vi "Get All Combinations.vi"(11 "Game Board in":refnum<class "Game Board.lvclass">) -> (3 "Game Board out":refnum<class "Game Board.lvclass">)   [LabVIEW 2024, in "Game Board.lvclass"]
doc: "MIT Licence\nCopyright (c) 2024 David Grollier"
uses:
  Game Board.lvclass
  Combinations Collision.ctl
  Collision/Collision.lvclass
  Game Board.lvclass/Game Board.ctl
  Game Board Component/Movable/Movable.lvclass
  Game Board Component/Game Board Component.lvclass
panel:
  out "appended array":string[][](array[string])
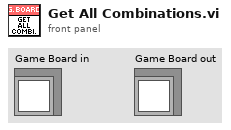
[diagram p1: front panel]
types:
  T1 = typedef "Game Board.lvclass/Combinations Collision.ctl" = cluster{"Collision":refnum<class "Collision.lvclass">, "Combination":string[]}
  T2 = map{string, refnum<class "Game Board Component.lvclass">}
  T3 = cluster{"Name":string, "Game Board Component":refnum<class "Game Board Component.lvclass">}[]
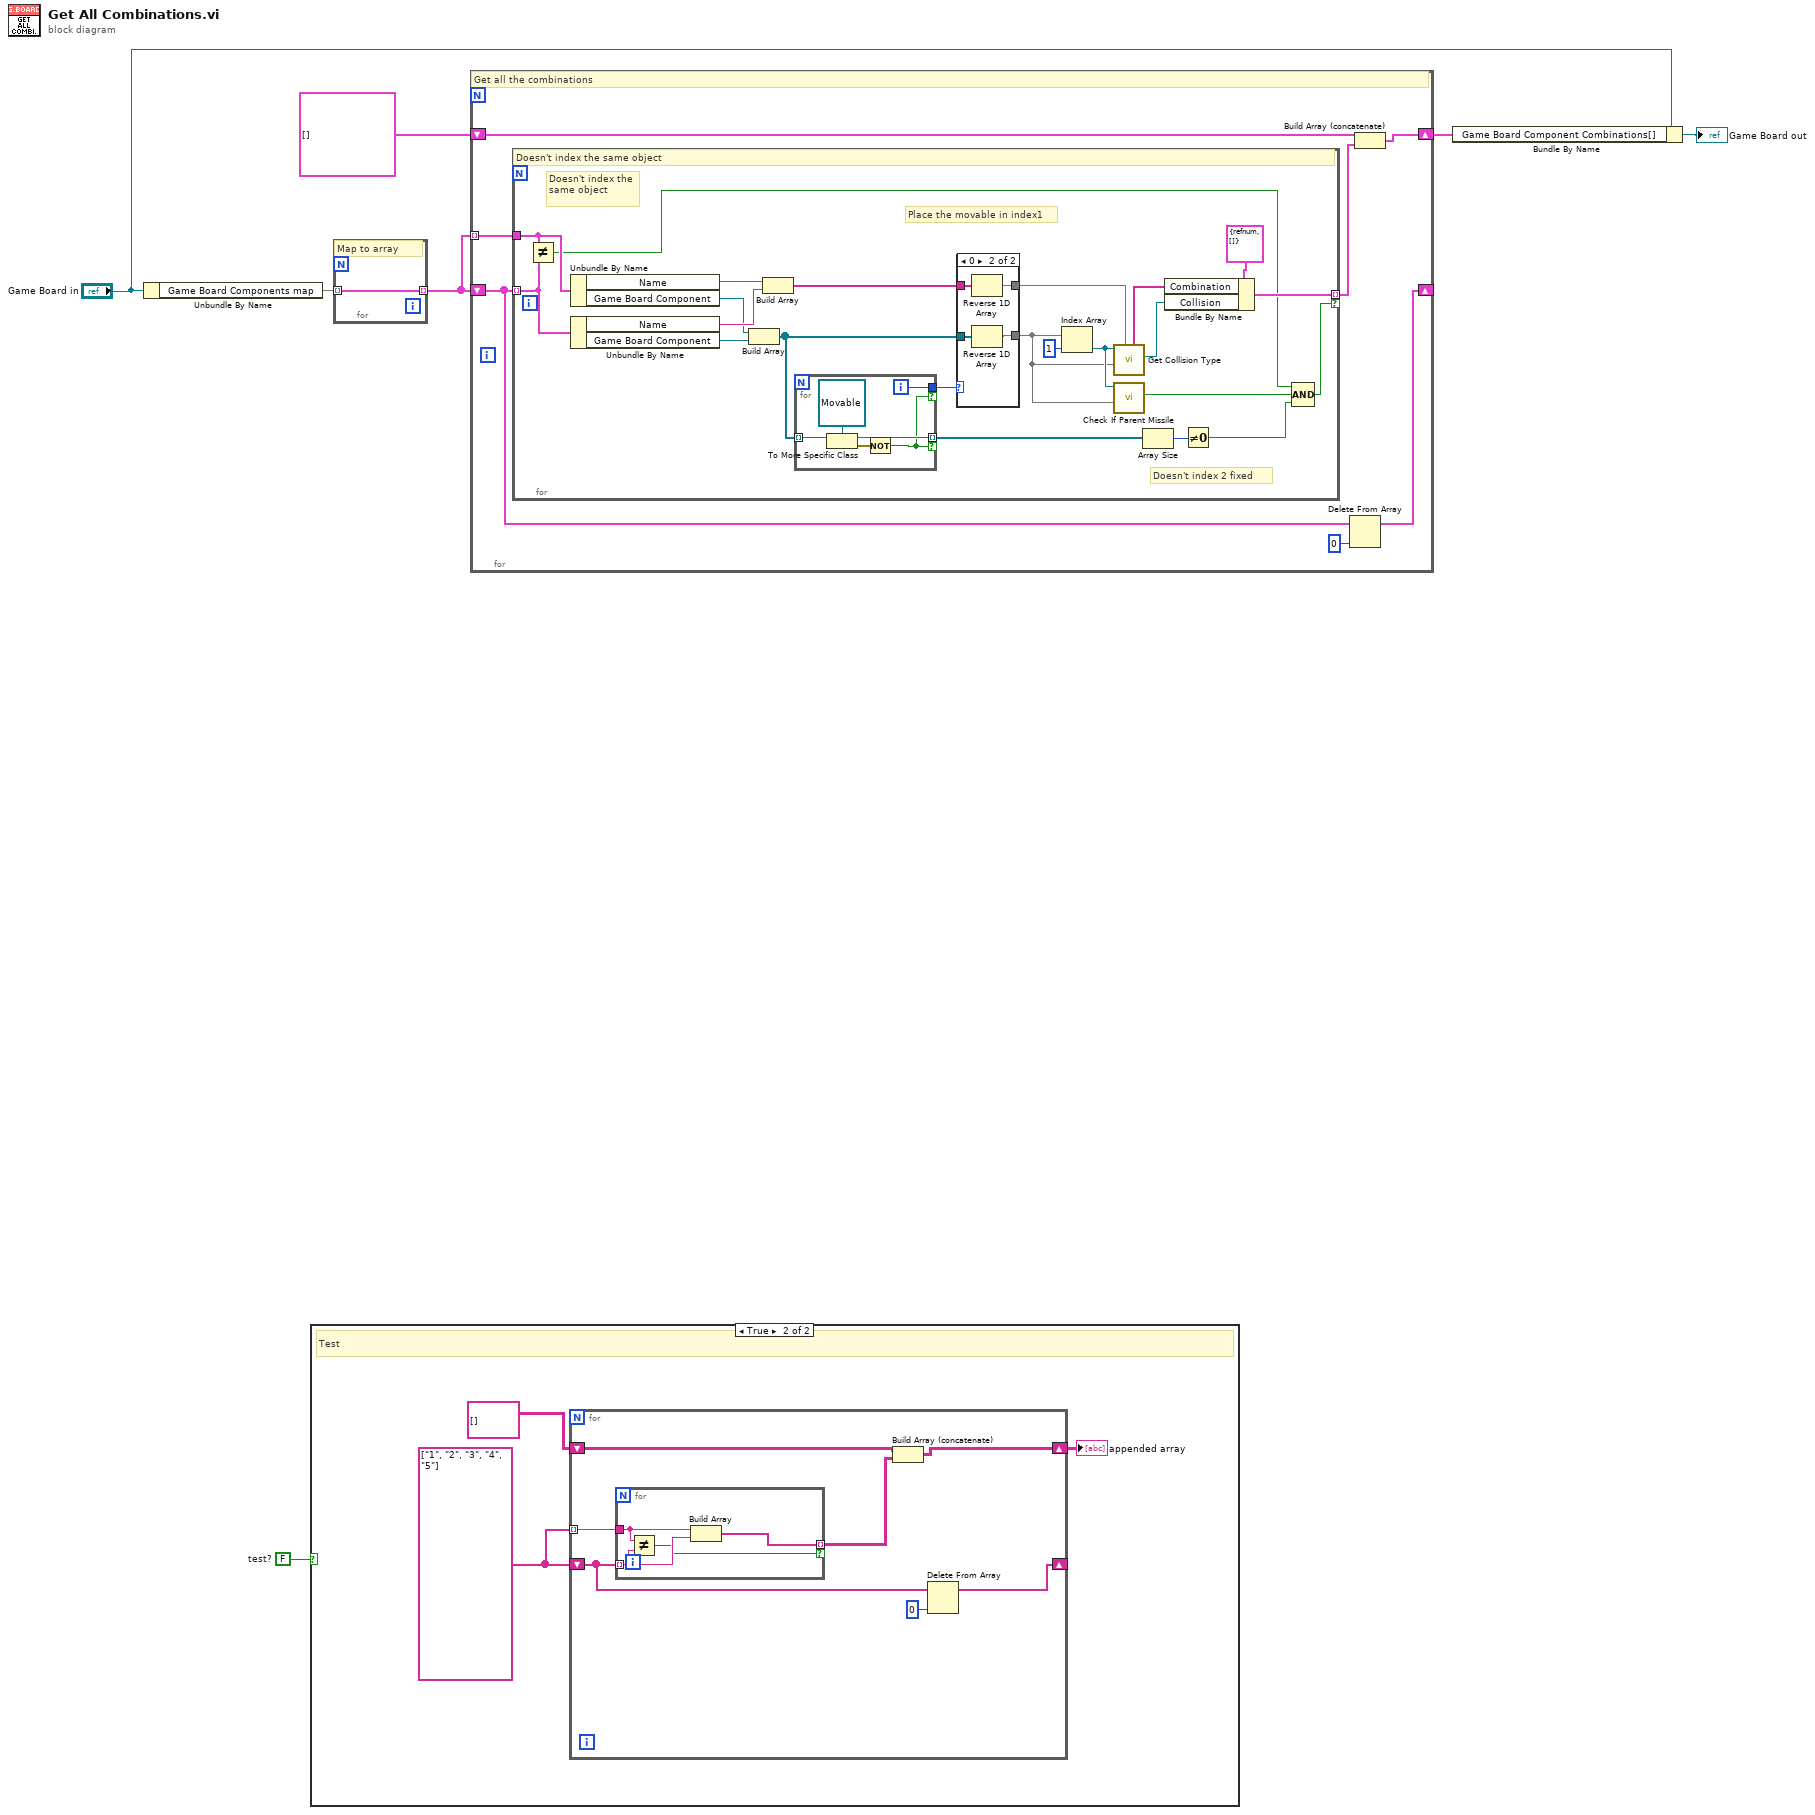
[diagram p0: block diagram]
diagram:
  w5 = FALSE  # test?
  n1 = Unbundle By Name("Game Board in") -> ("Game Board Components map"=w4:T2)
  n2 = case shown="True" w5 {
    frame False {
    }
    frame True {
      w8 = string[] ["1", "2", "3", "4", "5"]
      # "Test"
      n3 = for {
        tunnel: w8 -> [w17] mode=indexing
        shift-right: [w14] -> w10
        shift-left: string[][] [] ("appended array") -> [w15]
        shift-right: [w12] -> _
        shift-left: w8 -> [w13]
        n4 = for {
          tunnel: w13 -> [w19] mode=indexing
          tunnel: w17 -> [w20]
          tunnel: [w21] -> w16 mode=indexing if=w18
          n5 = Not Equal?(x=w20, y=w19) -> (x != y?=w18:bool)
          n6 = Build Array(w20, w19) -> (w21:string[])
        }
        n7 = Build Array (concatenate)(w15, w16) -> (w14:string[][])
        n8 = Delete From Array(array=w13, index=0) -> (array with subset deleted=w12:string[])  [unwired: 1 in, 1 out]
      }
      "appended array" <- w10
    }
  }
  n9 = for {
    tunnel: w4 -> [w22] mode=indexing
    tunnel: [w22] -> w1 mode=indexing
    # "Map to array"
  }
  n10 = for {
    tunnel: w1 -> [w29] mode=indexing
    shift-right: [w26] -> w2
    shift-left: T1[] [] -> [w27]
    shift-right: [w25] -> _
    shift-left: w1 -> [w23]
    # "Get all the combinations"
    n11 = for {
      tunnel: w23 -> [w47] mode=indexing
      tunnel: w29 -> [w49]
      tunnel: [w51] -> w28 mode=indexing if=w33
      # "Place the movable in index1"
      # "Doesn't index 2 fixed"
      # "Doesn't index the same object"
      # "Doesn't index the same object"
      n12 = Not Equal?(x=w49, y=w47) -> (x != y?=w31:bool)
      n13 = Unbundle By Name(w49) -> ("Name"=w48:string, "Game Board Component"=w45:refnum<class "Game Board Component.lvclass">)
      n14 = Unbundle By Name(w47) -> ("Name"=w46:string, "Game Board Component"=w44:refnum<class "Game Board Component.lvclass">)
      n15 = Build Array(w45, w44) -> (w40:refnum<class "Game Board Component.lvclass">[])
      n16 = Build Array(w48, w46) -> (w50:string[])
      n17 = for {
        tunnel: w40 -> [w57] mode=indexing
        tunnel: [w56] -> w43 mode=indexing if=w53
        tunnel: [w54] -> w41 if=w53
        i -> [w54]
        n18 = To More Specific Class(target class=refnum<class "Movable.lvclass"> refnum ("Movable.lvclass"), reference=w57) -> (specific class reference=w56:refnum<class "Movable.lvclass">, error out=w55:errorcluster)  [unwired: 1 in]
        n19 = Not(x=w55) -> (.not. x?=w53:bool)
      }
      n20 = case shown="0" w41 {
        tunnel: w50 -> [w60 w64]
        tunnel: [w60 w63] -> w37
        tunnel: w40 -> [w59 w62]
        tunnel: [w59 w61] -> w34
        frame Default {
        }
        frame 0 {
          n21 = Reverse 1D Array(array=w64) -> (reversed array=w63:string[])
          n22 = Reverse 1D Array(array=w62) -> (reversed array=w61:refnum<class "Game Board Component.lvclass">[])
        }
      }
      n23 = Index Array(array=w34, index=1) -> (element=w35:refnum<class "Game Board Component.lvclass">)
      n24 = call-dynamic "Get Collision Type.vi"("Combination in"=w37, "GB Components in"=w34, "Game Board Component in"=w35) -> ("Collision out"=w39:refnum<class "Collision.lvclass">, "Combination out"=w36:string[])  [unwired: 7 in]
      n25 = call-dynamic "Check If Parent Missile.vi"("GB Components in"=w34, "Game Board Component in"=w35) -> ("Not parent missile?"=w30:bool)  [unwired: 9 in]
      n26 = Array Size(array=w43) -> (size(s)=w42:i32)
      n27 = Bundle By Name(cluster=T1 {"Collision"=refnum, "Combination"=[]} ("Game Board Component Combinations[]"), "Combination"=w36, "Collision"=w39) -> (w51:T1)
      n28 = Not Equal To 0?(x=w42) -> (x != 0?=w32:bool)
      n29 = Compound Arithmetic op=AND(w31, w30, w32) -> (w33:bool)
    }
    n30 = Delete From Array(array=w23, index=0) -> (array with subset deleted=w25:T3)  [unwired: 1 in, 1 out]
    n31 = Build Array (concatenate)(w27, w28) -> (w26:T1[])
  }
  n32 = Bundle By Name(cluster="Game Board in", "Game Board Component Combinations[]"=w2) -> (→"Game Board out":refnum<class "Game Board.lvclass">)
